vi "getTRVendorPart.vi"(5 "RC No":string, 9 "Machine":string) -> (3 "Carrier":string, 4 "Width":dbl, 6 "Vendor":string, 10 "Cover":string, 13 "Time":i32, 14 "Temp":i32, 15 "PSI":dbl)   [LabVIEW 2012]
uses:
  <vilib>/addons/database/Connection.llb/DB Tools Open Connec (Path).vi
  <vilib>/addons/database/Connection.llb/Conn Execute.vi
  <vilib>/addons/database/Recordset.llb/Rec Fetch String Data (R).vi
  <vilib>/addons/database/Recordset.llb/Rec Destroy - Connection.vi
  <vilib>/addons/database/Recordset.llb/Rec Fetch Recordset Data (R).vi
  <vilib>/addons/database/_DB Variant To Data/Database Variant To Data.xnode
  <vilib>/addons/database/NI_Database_API.lvlib
panel:
  out "data 3":dbl
  out "data":string
  out "concatenated string 2":string
  out "WidthUnit":string
  out "concatenated string":string
  out "error out":errorcluster
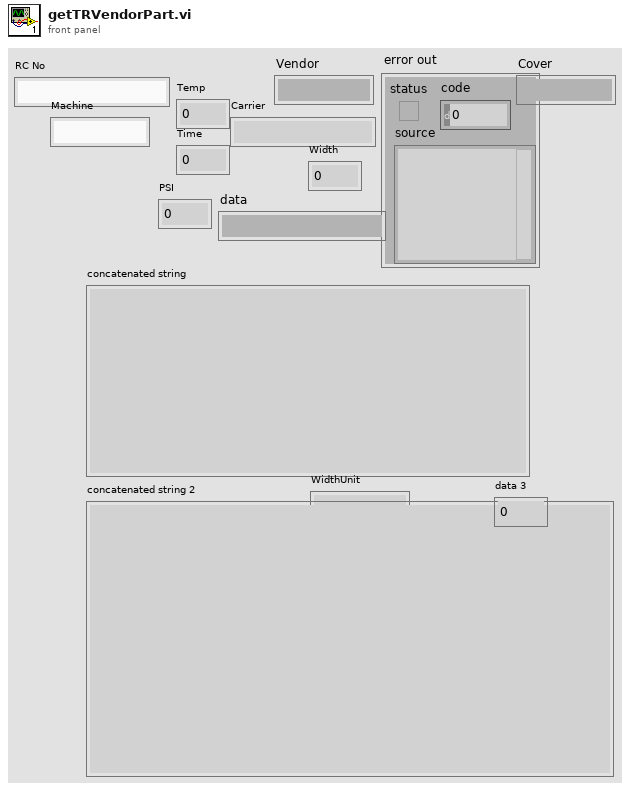
[diagram p1: front panel]
types:
  T1 = typedef "NI_Database_API.lvlib/Conn ObjectReference.ctl" = refnum<k1>
  T2 = typedef "NI_Database_API.lvlib/Rec ObjectReference.ctl" = refnum<k1>
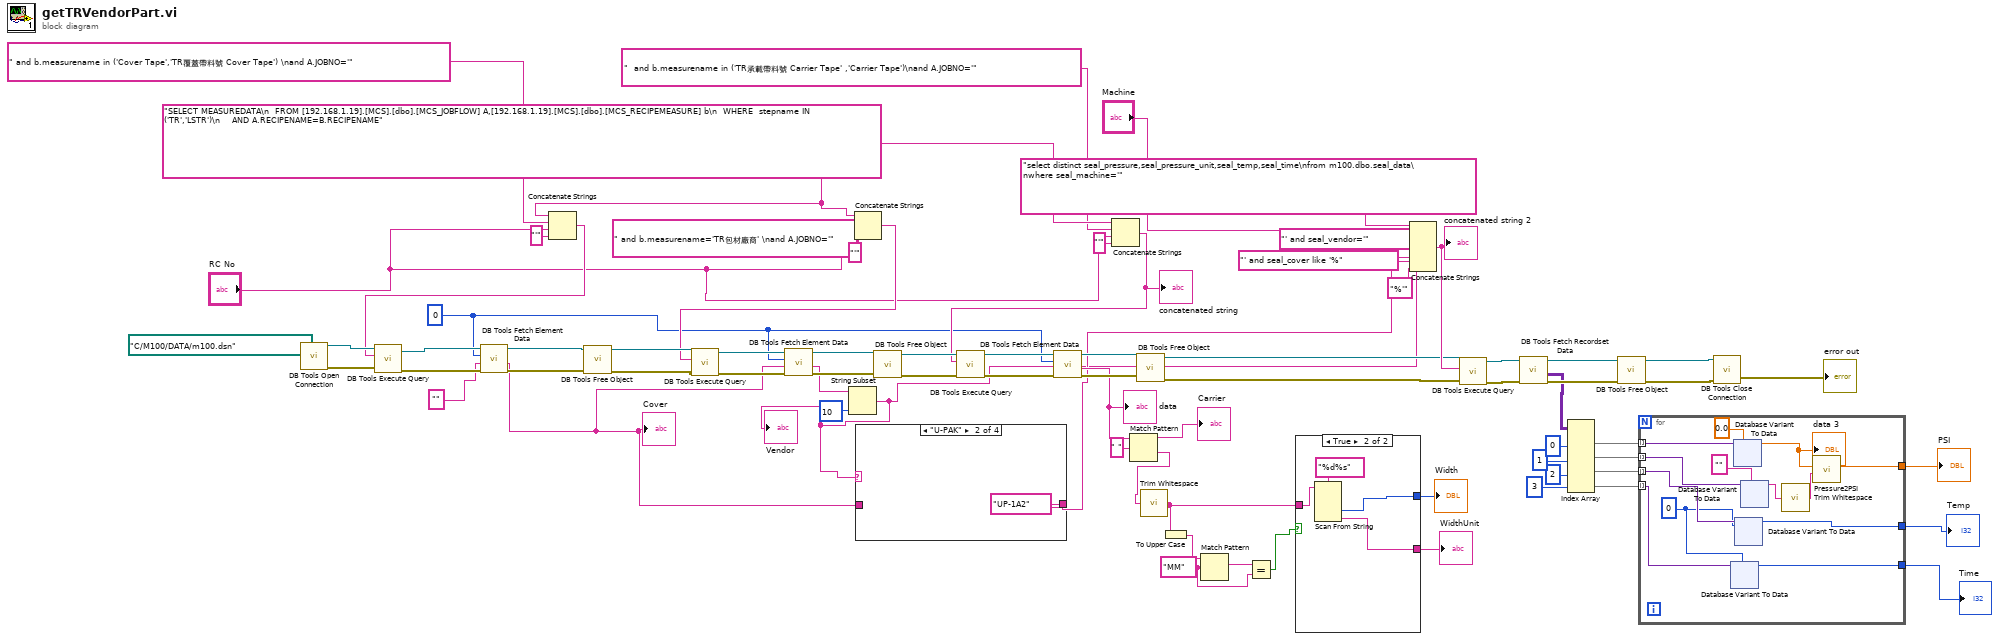
[diagram p0: block diagram]
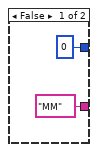
[diagram p2: hidden frame]
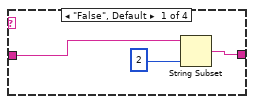
[diagram p3: hidden frame]
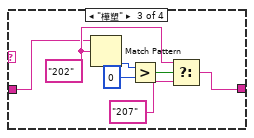
[diagram p4: hidden frame]
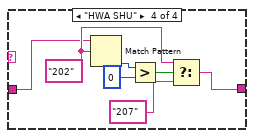
[diagram p5: hidden frame]
diagram:
  w8 = "MM" ("regular expression")
  w13 = 0
  w58 = "SELECT MEASUREDATA\n  FROM [192.168.1.19].[MCS].[dbo].[MCS_JOBFLOW] A,[192.168.1.19].[MCS].[dbo].[MCS_RECIPEMEASURE] b\n  WHERE  stepname IN ('TR','LSTR')\n    AND A.RECIPENAME=B.RECIPENAME" ("string")
  n1 = call-poly <vilib>:"DB Tools Open Connection.vi"("connection information"=path "C:/M100/DATA/m100.dsn") -> ("error out"=w71:errorcluster, "connection reference"=w73:T1)  [unwired: 7 in]
  n2 = Concatenate Strings(w58, " and b.measurename in ('Cover Tape','TR覆蓋帶料號 Cover Tape') \nand A.JOBNO='" ("string"), "RC No", "'" ("string")) -> (w44:string)
  n3 = call-poly <vilib>:"DB Tools Execute Query.vi"("error in (no error)"=w71, "SQL query"=w44, "connection reference"=w73) -> ("error out"=w70:errorcluster, "recordset reference"=w14:T2)  [unwired: 5 in]
  n4 = call-poly <vilib>:"DB Tools Fetch Element Data.vi"("error in (no error)"=w70, "type"="", "column index"=w13, "recordset reference"=w14) -> ("error out"=w69:errorcluster, "data"=w4:string, "recordset reference out"=w72:T2)  [unwired: 3 in]
  "Cover" <- w4
  n5 = call-poly <vilib>:"DB Tools Free Object.vi"("error in (no error)"=w69, "recordset reference"=w72) -> ("error out"=w63:errorcluster, "connection reference"=w66:T1)  [unwired: 8 in]
  n6 = Concatenate Strings(w58, " and b.measurename='TR包材廠商' \nand A.JOBNO='" ("string"), "RC No", "'" ("string")) -> (w56:string)
  n7 = call-poly <vilib>:"DB Tools Execute Query.vi"("error in (no error)"=w63, "SQL query"=w56, "connection reference"=w66) -> ("error out"=w62:errorcluster, "recordset reference"=w65:T2)  [unwired: 5 in]
  n8 = call-poly <vilib>:"DB Tools Fetch Element Data.vi"("error in (no error)"=w62, "type"=w4, "column index"=w13, "recordset reference"=w65) -> ("error out"=w61:errorcluster, "data"=w3:string, "recordset reference out"=w64:T2)  [unwired: 3 in]
  n9 = String Subset(string=w3, length (rest)=10 ("length (rest)")) -> (substring=w1:string)  [unwired: 1 in]
  "Vendor" <- w1
  n10 = case shown="\"U-PAK\"" w1 {
    tunnel: w4 -> [w78 _ w81 w88]
    tunnel: [w76 "UP-1A2" ("f") w80 w87] -> w36
    frame "False", Default {
      n11 = String Subset(string=w78, length (rest)=2 ("length (rest)")) -> (substring=w76:string)  [unwired: 1 in]
    }
    frame "U-PAK" {
    }
    frame "樺塑" {
      w85 = "202" ("regular expression")
      n12 = Match Pattern(string=w81, regular expression=w85) -> (offset past match=w82:i32)  [unwired: 1 in, 3 out]
      n13 = Greater?(x=w82, y=0) -> (0:w84:bool)
      n14 = Select(t=w85, s=w84, f="207") -> (s? t:f=w80:string)
    }
    frame "HWA SHU" {
      w92 = "202" ("regular expression")
      n15 = Match Pattern(string=w88, regular expression=w92) -> (offset past match=w89:i32)  [unwired: 1 in, 3 out]
      n16 = Greater?(x=w89, y=0) -> (0:w91:bool)
      n17 = Select(t=w92, s=w91, f="207") -> (s? t:f=w87:string)
    }
  }
  n18 = call-poly <vilib>:"DB Tools Free Object.vi"("error in (no error)"=w61, "recordset reference"=w64) -> ("error out"=w53:errorcluster, "connection reference"=w54:T1)  [unwired: 8 in]
  n19 = Concatenate Strings(w58, "  and b.measurename in ('TR承載帶料號 Carrier Tape' ,'Carrier Tape')\nand A.JOBNO='" ("string"), "RC No", "'" ("string")) -> (w48:string)
  "concatenated string" <- w48
  n20 = call-poly <vilib>:"DB Tools Execute Query.vi"("error in (no error)"=w53, "SQL query"=w48, "connection reference"=w54) -> ("error out"=w50:errorcluster, "recordset reference"=w52:T2)  [unwired: 5 in]
  n21 = call-poly <vilib>:"DB Tools Fetch Element Data.vi"("error in (no error)"=w50, "type"=w1, "column index"=w13, "recordset reference"=w52) -> ("error out"=w49:errorcluster, "data"=w47:string, "recordset reference out"=w51:T2)  [unwired: 3 in]
  "data" <- w47
  n22 = Match Pattern(string=w47, regular expression=" ") -> (before substring=→"Carrier":string, after substring=w42:string)  [unwired: 1 in, 2 out]
  n23 = call-poly <vilib>:"DB Tools Free Object.vi"("error in (no error)"=w49, "recordset reference"=w51) -> ("error out"=w33:errorcluster, "connection reference"=w34:T1)  [unwired: 8 in]
  n24 = call <vilib>:"Trim Whitespace.vi"("string"=w42) -> ("trimmed string"=w11:string)  [unwired: 1 in]
  n25 = To Upper Case(1:w11) -> (0:w10:string)
  n26 = Match Pattern(string=w10, regular expression=w8) -> (match substring=w9:string)  [unwired: 1 in, 3 out]
  n27 = Equal?(x=w9, y=w8) -> (x = y?=w7:bool)
  n28 = case shown="True" w7 {
    tunnel: w11 -> [_ w98]
    tunnel: [0 w97] -> w6
    tunnel: ["MM" w96] -> w5
    frame False {
    }
    frame True {
      n29 = Scan From String(format string="%d%s", input string=w98) -> (output 1=w97:i32, output 2=w96:string)  [unwired: 4 in, 3 out]
    }
  }
  "Width" <- w6
  "WidthUnit" <- w5
  n30 = Concatenate Strings("select distinct seal_pressure,seal_pressure_unit,seal_temp,seal_time\nfrom m100.dbo.seal_data\nwhere seal_machine='" ("string"), "Machine", "' and seal_vendor='" ("string"), w1, "' and seal_cover like '%" ("string"), w36, "%'" ("string")) -> (w35:string)
  "concatenated string 2" <- w35
  n31 = call-poly <vilib>:"DB Tools Execute Query.vi"("error in (no error)"=w33, "SQL query"=w35, "connection reference"=w34) -> ("error out"=w31:errorcluster, "recordset reference"=w32:T2)  [unwired: 5 in]
  n32 = call-poly <vilib>:"DB Tools Fetch Recordset Data.vi"("error in (no error)"=w31, "recordset reference"=w32) -> ("error out"=w29:errorcluster, "recordset data"=w26:variant[][], "recordset reference out"=w30:T2)  [unwired: 3 in]
  n33 = Index Array(array=w26, index (col) #1=0 ("disabled index (col)"), index (col) #2=1 ("index (col)"), index (col) #3=2 ("index (col)"), index (col) #4=3 ("index (col)")) -> (element #1=w21:variant[], element #2=w20:variant[], element #3=w19:variant[], element #4=w18:variant[])  [unwired: 4 in]
  n34 = call-poly <vilib>:"DB Tools Free Object.vi"("error in (no error)"=w29, "recordset reference"=w30) -> ("error out"=w27:errorcluster, "connection reference"=w28:T1)  [unwired: 8 in]
  n35 = for {
    tunnel: w21 -> [w112] mode=indexing
    tunnel: w20 -> [w111] mode=indexing
    tunnel: w19 -> [w110] mode=indexing
    tunnel: w18 -> [w109] mode=indexing
    tunnel: [w104] -> w17
    tunnel: [w103] -> w16
    tunnel: [w102] -> w15
    w105 = 0
    n36 = xnode "Database Variant To Data"("database variant"=w109, "type"=w105) -> ("data"=w103:i32)  [unwired: 1 in, 1 out]
    n37 = xnode "Database Variant To Data"("database variant"=w112, "type"=0.0) -> ("data"=w106:dbl)  [unwired: 1 in, 1 out]
    "data 3" <- w106
    n38 = xnode "Database Variant To Data"("database variant"=w110, "type"=w105) -> ("data"=w104:i32)  [unwired: 1 in, 1 out]
    n39 = xnode "Database Variant To Data"("database variant"=w111, "type"="") -> ("data"=w101:string)  [unwired: 1 in, 1 out]
    n40 = call <vilib>:"Trim Whitespace.vi"("string"=w101) -> ("trimmed string"=w100:string)  [unwired: 1 in]
    n41 = call "Pressure2PSI.vi"("Unit"=w100, "Numeric"=w106) -> ("PSI"=w102:dbl)  [unwired: 9 in]
  }
  "Temp" <- w17
  "Time" <- w16
  "PSI" <- w15
  n42 = call <vilib>:"DB Tools Close Connection.vi"("error in (no error)"=w27, "connection reference"=w28) -> ("error out"=→"error out":errorcluster)  [unwired: 5 in]
